vi "Pierwsze zajęcia z LabView 02.10.20.vi"() -> ()   [LabVIEW 2020]
panel:
  out "Czy Pitagorejski?":bool
  out "Czy trojkat?":bool
  out "S":dbl
  in  "C":dbl
  in  "B":dbl
  in  "A":dbl
  out "Sekundy":dbl
  out "Minuty":dbl
  out "Godziny\nGodziny":dbl
  in  "czas w sekundach":dbl
  out "XOR":bool
  out "NOT A":bool
  out "OR\nOR\nOR":bool
  out "AND":bool
  in  "Boolean":bool
  in  "Boolean 2":bool
  out "x+y":dbl
  out "x .and. y?":bool
  out "A+B":dbl
  in  "B\n4":dbl
  in  "A":dbl
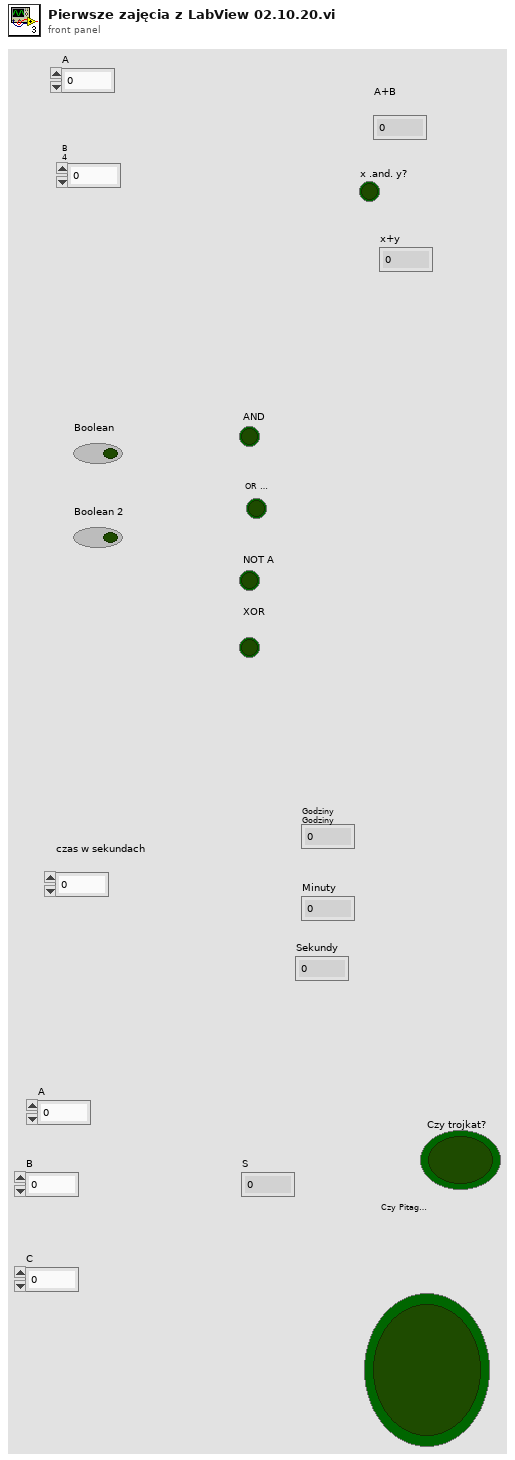
[diagram p1: front panel]
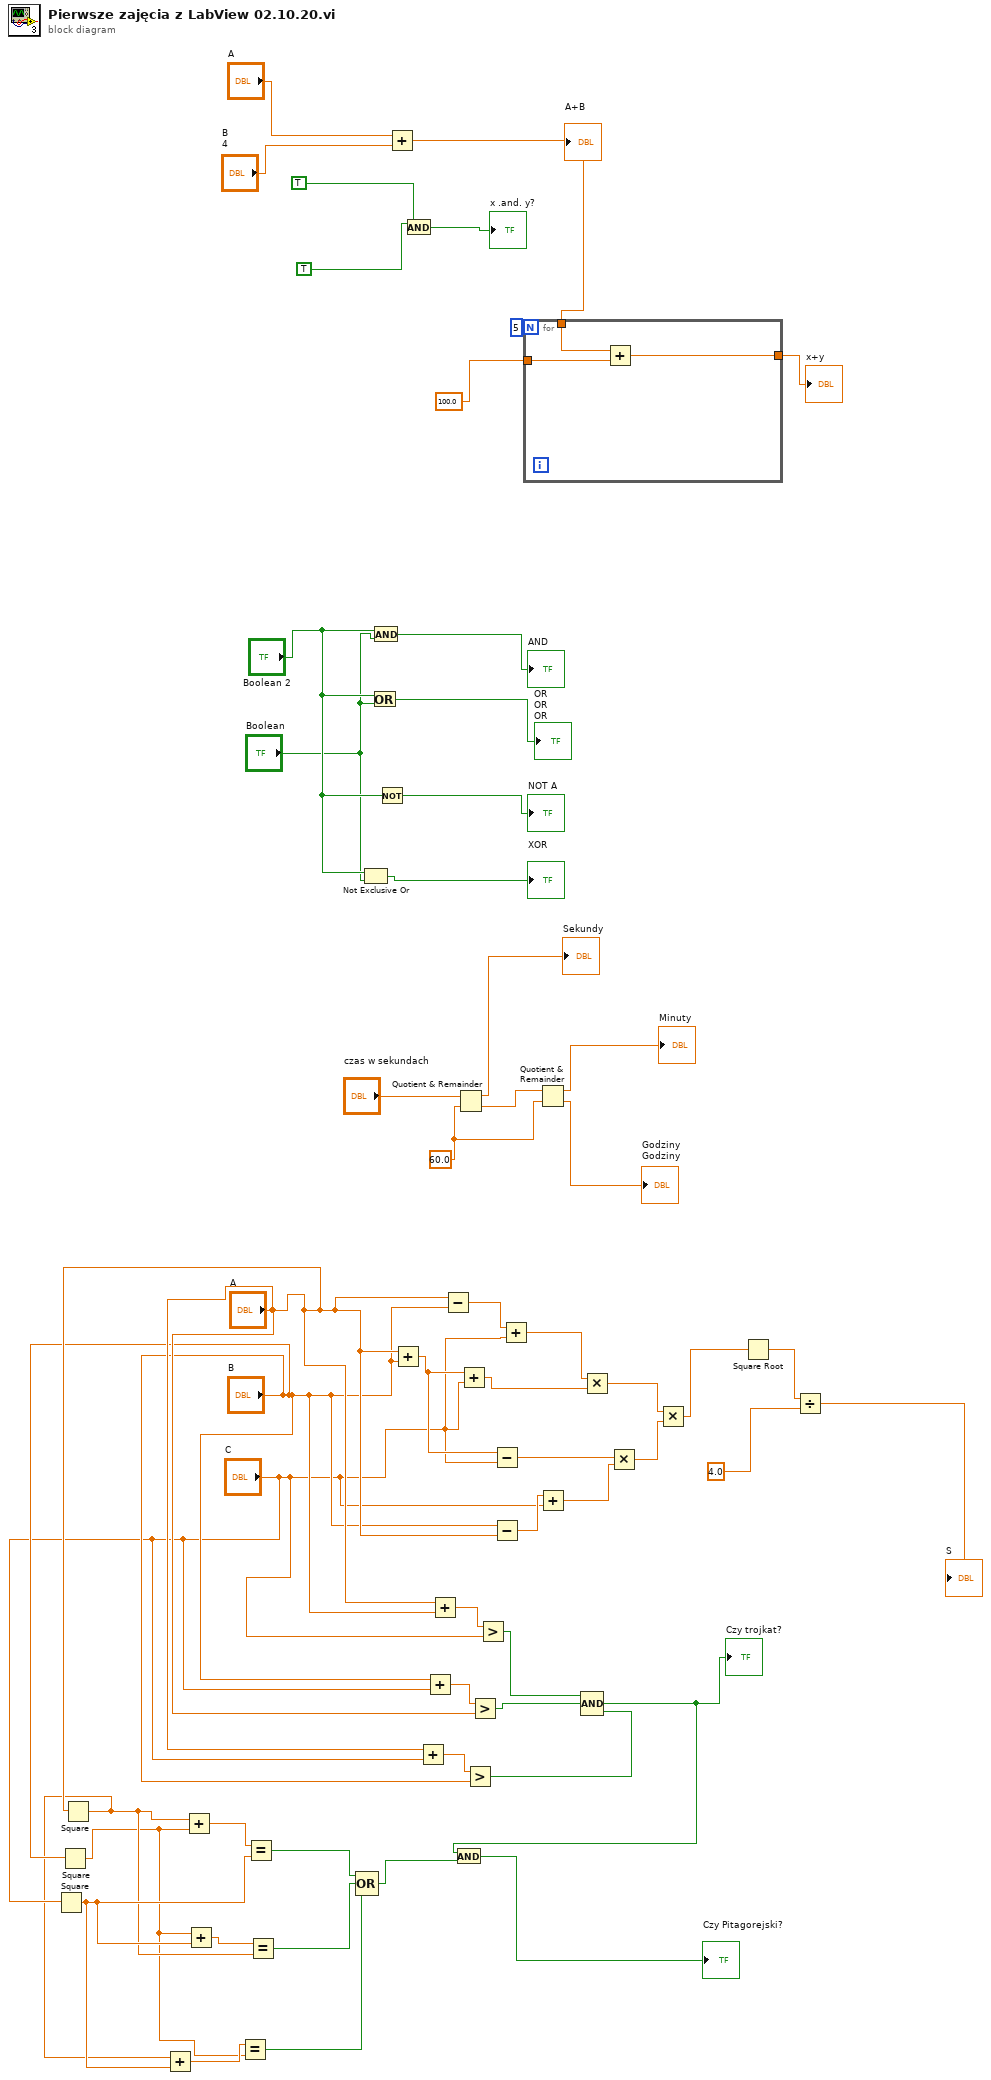
[diagram p0: block diagram]
diagram:
  w38 = 60.0
  n1 = Square(x="C") -> (x^2=w10:dbl)
  n2 = Square(x="B") -> (x^2=w5:dbl)
  n3 = Square(x="A") -> (x^2=w8:dbl)
  n4 = Add(x=w8, y=w10) -> (x+y=w6:dbl)
  n5 = Add(x=w8, y=w5) -> (x+y=w12:dbl)
  n6 = Add(x=w5, y=w10) -> (x+y=w9:dbl)
  n7 = Equal?(x=w6, y=w5) -> (x = y?=w4:bool)
  n8 = Equal?(x=w12, y=w10) -> (x = y?=w11:bool)
  n9 = Equal?(x=w9, y=w8) -> (x = y?=w7:bool)
  n10 = Compound Arithmetic op=OR(w11, w7, w4) -> (w2:bool)
  n11 = Not Exclusive Or(1:"Boolean", 2:"Boolean 2") -> (0:→"XOR":bool)
  n12 = Or(x="Boolean 2", y="Boolean") -> (x .or. y?=→"OR\nOR\nOR":bool)
  n13 = And(x="Boolean 2", y="Boolean") -> (x .and. y?=→"AND":bool)
  n14 = Not(x="Boolean 2") -> (.not. x?=→"NOT A":bool)
  n15 = Add(x="A", y="B\n4") -> (x+y=w50:dbl)
  "A+B" <- w50
  n16 = Add(x="A", y="B") -> (x+y=w34:dbl)
  n17 = And(x=TRUE ("y"), y=TRUE) -> (x .and. y?=→"x .and. y?":bool)
  n18 = Add(x="A", y="C") -> (x+y=w19:dbl)
  n19 = Add(x="B", y="C") -> (x+y=w20:dbl)
  n20 = Add(x="A", y="B") -> (x+y=w21:dbl)
  n21 = Subtract(x="A", y="B") -> (x-y=w33:dbl)
  n22 = Quotient & Remainder(x="czas w sekundach", y=w38) -> (x-y*floor(x/y)=→"Sekundy":dbl, floor(x/y)=w37:dbl)
  n23 = Add(x=w34, y="C") -> (x+y=w30:dbl)
  n24 = Greater?(x=w19, y="B") -> (0:w16:bool)
  n25 = Greater?(x=w20, y="A") -> (0:w17:bool)
  n26 = Greater?(x=w21, y="C") -> (0:w18:bool)
  n27 = Subtract(x=w34, y="C") -> (x-y=w29:dbl)
  n28 = Subtract(x="B", y="A") -> (x-y=w32:dbl)
  n29 = Add(x=w33, y="C") -> (x+y=w31:dbl)
  n30 = for {
    N: 5 -> [_]
    tunnel: w50 -> [w58]
    tunnel: 100.0 ("x+y") -> [w57]
    tunnel: [w56] -> w47
    n31 = Add(x=w58, y=w57) -> (x+y=w56:dbl)
  }
  "x+y" <- w47
  n32 = Quotient & Remainder(x=w37, y=w38) -> (x-y*floor(x/y)=→"Minuty":dbl, floor(x/y)=→"Godziny\nGodziny":dbl)
  n33 = Add(x=w32, y="C") -> (x+y=w28:dbl)
  n34 = Compound Arithmetic op=AND(w18, w17, w16) -> (w3:bool)
  "Czy trojkat?" <- w3
  n35 = And(x=w3, y=w2) -> (x .and. y?=→"Czy Pitagorejski?":bool)
  n36 = Multiply(x=w31, y=w30) -> (x*y=w27:dbl)
  n37 = Multiply(x=w29, y=w28) -> (x*y=w26:dbl)
  n38 = Multiply(x=w27, y=w26) -> (x*y=w23:dbl)
  n39 = Square Root(x=w23) -> (sqrt(x)=w22:dbl)
  n40 = Divide(x=w22, y=4.0) -> (x/y=→"S":dbl)
